vi "Tosca-Read TTL Outputs.vi"(0 "Connection File Path thru":path, 11 "error in (no error)":errorcluster) -> (4 "Devices":refnum<class "TTLControlledDevice.lvclass">[](array[class]), 15 "error out":errorcluster)   [LabVIEW 2020]
uses:
  TTL VIs/Device Classes/Base Class/TTLControlledDevice.lvclass
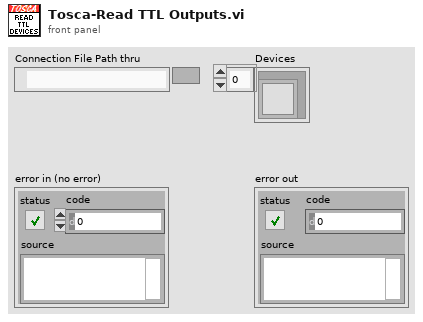
[diagram p1: front panel]
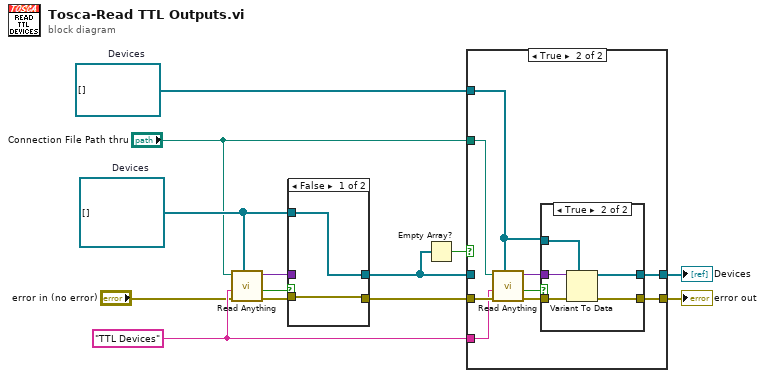
[diagram p0: block diagram]
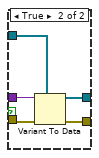
[diagram p2: hidden frame]
diagram:
  w13 = refnum<class "TTLControlledDevice.lvclass">[] []  # Devices
  w3 = refnum<class "TTLControlledDevice.lvclass">[] []  # Devices
  w12 = "TTL Devices" ("Section Name (Name of \"Type of Anything\")")
  n1 = call "Read Anything.vi"("Type of Anything"=w3, "Error In"="error in (no error)", "Section Name (Name of \"Type of Anything\")"=w12, "Path (dialog)"="Connection File Path thru") -> ("Error Out"=w7:errorcluster, "Found?"=w4:bool, "Anything"=w5:variant)  [unwired: 5 in]
  n2 = case shown="False" w4 {
    tunnel: w7 -> [w15 w20]
    tunnel: [w15 w19] -> w6
    tunnel: w5 -> [_ w18]
    tunnel: w3 -> [w14 w17]
    tunnel: [w14 w16] -> w2
    frame False {
    }
    frame True {
      n3 = Variant To Data(error in=w20, type=w17, Variant=w18) -> (data=w16:refnum<class "TTLControlledDevice.lvclass">[], error out=w19:errorcluster)
    }
  }
  n4 = Empty Array?(array=w2) -> (empty?=w9:bool)
  n5 = case shown="True" w9 {
    tunnel: [w22 w25] -> w11
    tunnel: w2 -> [w22 _]
    tunnel: w6 -> [w21 w31]
    tunnel: [w21 w24] -> w10
    tunnel: w13 -> [_ w26]
    tunnel: w12 -> [_ w29]
    tunnel: "Connection File Path thru" -> [_ w23]
    frame False {
    }
    frame True {
      n6 = call "Read Anything.vi"("Type of Anything"=w26, "Error In"=w31, "Section Name (Name of \"Type of Anything\")"=w29, "Path (dialog)"=w23) -> ("Error Out"=w27:errorcluster, "Found?"=w28:bool, "Anything"=w30:variant)  [unwired: 5 in]
      n7 = case shown="True" w28 {
        tunnel: w27 -> [w32 w38]
        tunnel: w30 -> [_ w37]
        tunnel: w26 -> [w33 w36]
        tunnel: [w33 w35] -> w25
        tunnel: [w32 w34] -> w24
        frame False {
        }
        frame True {
          n8 = Variant To Data(error in=w38, type=w36, Variant=w37) -> (data=w35:refnum<class "TTLControlledDevice.lvclass">[], error out=w34:errorcluster)
        }
      }
    }
  }
  "Devices" <- w11
  "error out" <- w10
